vi "Decode scancodes into ascii.vi"(2 "PlatMods":T1, 3 "Mods":cluster{"Num Pad":bool, "Menu Key":bool}, 4 "ScanCode":i16) -> (0 "Numeric":i16, 1 "String":string)   [LabVIEW 2013]
doc: "Decode scanscodes into ascii.vi takes the scancode, mods, and platmods to index a case structure that outputs the ASCII value and the numeric value of the ASCII. Use this VI in the key up event if you want to programatically capture keystrikes.\n\nThe VI is easy to use, but tedious to write. There are 93 cases, each of which was experimentally verified."
panel:
  # "Select Help»Show Context Help and move the cursor \nover the VI icon to display help for this VI."
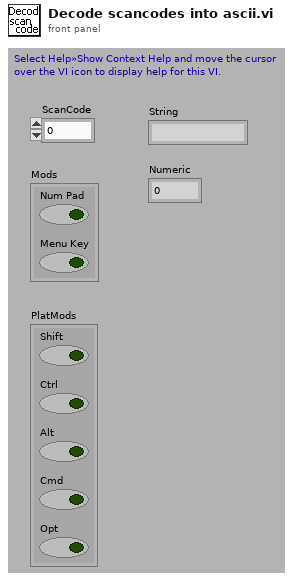
[diagram p1: front panel]
types:
  T1 = cluster{"Shift":bool, "Ctrl":bool, "Alt":bool, "Cmd":bool, "Opt":bool}
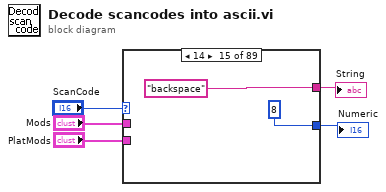
[diagram p0: block diagram]
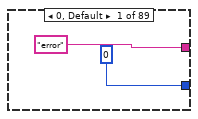
[diagram p2: hidden frame]
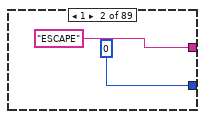
[diagram p3: hidden frame]
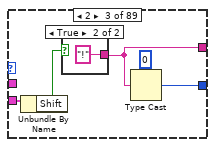
[diagram p4: hidden frame]
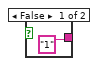
[diagram p5: hidden frame]
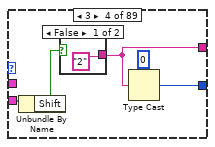
[diagram p6: hidden frame]
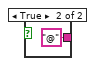
[diagram p7: hidden frame]
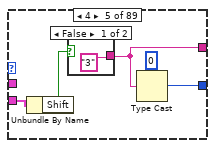
[diagram p8: hidden frame]
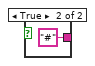
[diagram p9: hidden frame]
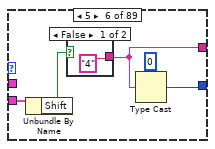
[diagram p10: hidden frame]
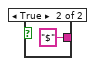
[diagram p11: hidden frame]
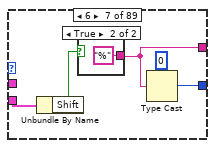
[diagram p12: hidden frame]
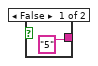
[diagram p13: hidden frame]
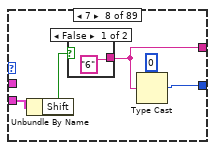
[diagram p14: hidden frame]
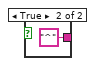
[diagram p15: hidden frame]
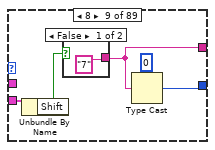
[diagram p16: hidden frame]
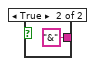
[diagram p17: hidden frame]
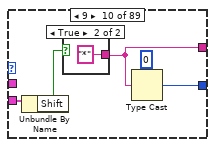
[diagram p18: hidden frame]
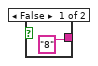
[diagram p19: hidden frame]
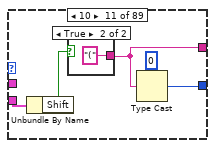
[diagram p20: hidden frame]
diagram:
  n1 = case shown="14" "ScanCode" {
    tunnel: ["error" "ESCAPE" w11 w19 w27 w35 w41 w45 w56 w63 w70 w76 w82 w87 "backspace" "tab" w100 w107 w114 w119 w126 w133 w140 w147 w154 w161 w168 w175 "Enter" "control" w188 w194 w202 w208 w215 w222 w229 w236 w243 w250 w256 w263 w272 w274 w282 w288 w295 w301 w308 w315 w322 w329 w336 w344 "RSHIFT" w355 "RSHIFT" "SPACE" "CAPSLOCK" "F1" "F2" "F3" "F4" "F5" "F6" "F7" "F8" "F9" "F10" "numlock" w389 w394 w403 w410 w419 w423 w431 w435 w443 w447 w455 w465 w476 w485 w491 w495 "left win key" "right win key" "select"] -> w2
    tunnel: "Mods" -> [_ _ _ _ _ _ _ _ _ _ _ _ _ _ _ _ _ _ _ _ _ _ _ _ _ _ _ _ _ _ _ _ _ _ _ _ _ _ _ _ _ _ _ _ _ _ _ _ _ _ _ _ _ _ _ w352 _ _ _ _ _ _ _ _ _ _ _ _ _ _ _ w393 w402 w412 _ w424 _ w436 _ w448 w457 w466 w473 w482 _ _ _ _ _]
    tunnel: "PlatMods" -> [_ _ w12 w18 w24 w32 w38 w47 w53 w60 w67 w73 w80 w89 _ _ w98 w105 w112 w120 w128 w134 w141 w149 w156 w163 w170 w177 _ _ w186 w193 w200 w207 w214 w221 w228 w235 w242 w249 w257 w264 _ w273 w283 w287 w294 w302 w309 w316 w323 w330 w337 w343 _ _ _ _ _ _ _ _ _ _ _ _ _ _ _ _ _ _ _ _ _ _ _ _ _ _ _ _ _ _ _ _ _ _ _]
    tunnel: [u8 0 u8 0 w13 w17 w28 w31 w42 w46 w52 w59 w66 w77 w81 w88 u8 8 u8 9 w99 w106 w113 w123 w127 w137 w144 w148 w155 w162 w169 w176 u8 0 u8 0 w187 w197 w201 w211 w218 w225 w232 w239 w246 w253 w260 w267 w270 w277 w281 w291 w298 w305 w312 w319 w326 w333 w340 w347 u8 0 w354 u8 0 u8 32 u8 0 u8 0 u8 0 u8 0 u8 0 u8 0 u8 0 u8 0 u8 0 u8 0 u8 0 u8 0 w390 w392 w404 w411 w420 w422 w432 w434 w444 w446 w456 w464 w475 w484 w492 w494 u8 0 u8 0 u8 0] -> w5
    frame 0, Default {
    }
    frame 1 {
    }
    frame 2 {
      n2 = Unbundle By Name(w12) -> ("Shift"=w10:bool)
      n3 = case shown="True" w10 {
        tunnel: ["1" "!"] -> w11
        frame False {
        }
        frame True {
        }
      }
      n4 = Type Cast(type=u8 0, x=w11) -> (*(type *) &x=w13:u8)
    }
    frame 3 {
      n5 = Unbundle By Name(w18) -> ("Shift"=w20:bool)
      n6 = case shown="False" w20 {
        tunnel: ["2" "@"] -> w19
        frame False {
        }
        frame True {
        }
      }
      n7 = Type Cast(type=u8 0, x=w19) -> (*(type *) &x=w17:u8)
    }
    frame 4 {
      n8 = Unbundle By Name(w24) -> ("Shift"=w25:bool)
      n9 = case shown="False" w25 {
        tunnel: ["3" "#"] -> w27
        frame False {
        }
        frame True {
        }
      }
      n10 = Type Cast(type=u8 0, x=w27) -> (*(type *) &x=w28:u8)
    }
    frame 5 {
      n11 = Unbundle By Name(w32) -> ("Shift"=w33:bool)
      n12 = case shown="False" w33 {
        tunnel: ["4" "$"] -> w35
        frame False {
        }
        frame True {
        }
      }
      n13 = Type Cast(type=u8 0, x=w35) -> (*(type *) &x=w31:u8)
    }
    frame 6 {
      n14 = Unbundle By Name(w38) -> ("Shift"=w39:bool)
      n15 = case shown="True" w39 {
        tunnel: ["5" "%"] -> w41
        frame False {
        }
        frame True {
        }
      }
      n16 = Type Cast(type=u8 0, x=w41) -> (*(type *) &x=w42:u8)
    }
    frame 7 {
      n17 = Unbundle By Name(w47) -> ("Shift"=w49:bool)
      n18 = case shown="False" w49 {
        tunnel: ["6" "^"] -> w45
        frame False {
        }
        frame True {
        }
      }
      n19 = Type Cast(type=u8 0, x=w45) -> (*(type *) &x=w46:u8)
    }
    frame 8 {
      n20 = Unbundle By Name(w53) -> ("Shift"=w55:bool)
      n21 = case shown="False" w55 {
        tunnel: ["7" "&"] -> w56
        frame False {
        }
        frame True {
        }
      }
      n22 = Type Cast(type=u8 0, x=w56) -> (*(type *) &x=w52:u8)
    }
    frame 9 {
      n23 = Unbundle By Name(w60) -> ("Shift"=w61:bool)
      n24 = case shown="True" w61 {
        tunnel: ["8" "*"] -> w63
        frame False {
        }
        frame True {
        }
      }
      n25 = Type Cast(type=u8 0, x=w63) -> (*(type *) &x=w59:u8)
    }
    frame 10 {
      n26 = Unbundle By Name(w67) -> ("Shift"=w69:bool)
      n27 = case shown="True" w69 {
        tunnel: ["9" "("] -> w70
        frame False {
        }
        frame True {
        }
      }
      n28 = Type Cast(type=u8 0, x=w70) -> (*(type *) &x=w66:u8)
    }
    frame 11 {
      n29 = Unbundle By Name(w73) -> ("Shift"=w74:bool)
      n30 = case shown="False" w74 {
        tunnel: ["0" ")"] -> w76
        frame False {
        }
        frame True {
        }
      }
      n31 = Type Cast(type=u8 0, x=w76) -> (*(type *) &x=w77:u8)
    }
    frame 12 {
      n32 = Unbundle By Name(w80) -> ("Shift"=w84:bool)
      n33 = case shown="False" w84 {
        tunnel: ["-" "_"] -> w82
        frame False {
        }
        frame True {
        }
      }
      n34 = Type Cast(type=u8 0, x=w82) -> (*(type *) &x=w81:u8)
    }
    frame 13 {
      n35 = Unbundle By Name(w89) -> ("Shift"=w90:bool)
      n36 = case shown="False" w90 {
        tunnel: ["=" "+"] -> w87
        frame False {
        }
        frame True {
        }
      }
      n37 = Type Cast(type=u8 0, x=w87) -> (*(type *) &x=w88:u8)
    }
    frame 14 {
    }
    frame 15 {
    }
    frame 16 {
      n38 = Unbundle By Name(w98) -> ("Shift"=w102:bool)
      n39 = case shown="True" w102 {
        tunnel: ["q" "Q"] -> w100
        frame False {
        }
        frame True {
        }
      }
      n40 = Type Cast(type=u8 0, x=w100) -> (*(type *) &x=w99:u8)
    }
    frame 17 {
      n41 = Unbundle By Name(w105) -> ("Shift"=w108:bool)
      n42 = case shown="True" w108 {
        tunnel: ["w" "W"] -> w107
        frame False {
        }
        frame True {
        }
      }
      n43 = Type Cast(type=u8 0, x=w107) -> (*(type *) &x=w106:u8)
    }
    frame 18 {
      n44 = Unbundle By Name(w112) -> ("Shift"=w116:bool)
      n45 = case shown="True" w116 {
        tunnel: ["e" "E"] -> w114
        frame False {
        }
        frame True {
        }
      }
      n46 = Type Cast(type=u8 0, x=w114) -> (*(type *) &x=w113:u8)
    }
    frame 19 {
      n47 = Unbundle By Name(w120) -> ("Shift"=w121:bool)
      n48 = case shown="True" w121 {
        tunnel: ["r" "R"] -> w119
        frame False {
        }
        frame True {
        }
      }
      n49 = Type Cast(type=u8 0, x=w119) -> (*(type *) &x=w123:u8)
    }
    frame 20 {
      n50 = Unbundle By Name(w128) -> ("Shift"=w129:bool)
      n51 = case shown="True" w129 {
        tunnel: ["t" "T"] -> w126
        frame False {
        }
        frame True {
        }
      }
      n52 = Type Cast(type=u8 0, x=w126) -> (*(type *) &x=w127:u8)
    }
    frame 21 {
      n53 = Unbundle By Name(w134) -> ("Shift"=w135:bool)
      n54 = case shown="True" w135 {
        tunnel: ["y" "Y"] -> w133
        frame False {
        }
        frame True {
        }
      }
      n55 = Type Cast(type=u8 0, x=w133) -> (*(type *) &x=w137:u8)
    }
    frame 22 {
      n56 = Unbundle By Name(w141) -> ("Shift"=w143:bool)
      n57 = case shown="True" w143 {
        tunnel: ["u" "U"] -> w140
        frame False {
        }
        frame True {
        }
      }
      n58 = Type Cast(type=u8 0, x=w140) -> (*(type *) &x=w144:u8)
    }
    frame 23 {
      n59 = Unbundle By Name(w149) -> ("Shift"=w150:bool)
      n60 = case shown="True" w150 {
        tunnel: ["i" "I"] -> w147
        frame False {
        }
        frame True {
        }
      }
      n61 = Type Cast(type=u8 0, x=w147) -> (*(type *) &x=w148:u8)
    }
    frame 24 {
      n62 = Unbundle By Name(w156) -> ("Shift"=w158:bool)
      n63 = case shown="True" w158 {
        tunnel: ["o" "O"] -> w154
        frame False {
        }
        frame True {
        }
      }
      n64 = Type Cast(type=u8 0, x=w154) -> (*(type *) &x=w155:u8)
    }
    frame 25 {
      n65 = Unbundle By Name(w163) -> ("Shift"=w165:bool)
      n66 = case shown="True" w165 {
        tunnel: ["p" "P"] -> w161
        frame False {
        }
        frame True {
        }
      }
      n67 = Type Cast(type=u8 0, x=w161) -> (*(type *) &x=w162:u8)
    }
    frame 26 {
      n68 = Unbundle By Name(w170) -> ("Shift"=w171:bool)
      n69 = case shown="True" w171 {
        tunnel: ["[" "{"] -> w168
        frame False {
        }
        frame True {
        }
      }
      n70 = Type Cast(type=u8 0, x=w168) -> (*(type *) &x=w169:u8)
    }
    frame 27 {
      n71 = Unbundle By Name(w177) -> ("Shift"=w179:bool)
      n72 = case shown="False" w179 {
        tunnel: ["}" "P"] -> w175
        frame False {
        }
        frame True {
        }
      }
      n73 = Type Cast(type=u8 0, x=w175) -> (*(type *) &x=w176:u8)
    }
    frame 28 {
    }
    frame 29 {
    }
    frame 30 {
      n74 = Unbundle By Name(w186) -> ("Shift"=w189:bool)
      n75 = case shown="True" w189 {
        tunnel: ["a" "A"] -> w188
        frame False {
        }
        frame True {
        }
      }
      n76 = Type Cast(type=u8 0, x=w188) -> (*(type *) &x=w187:u8)
    }
    frame 31 {
      n77 = Unbundle By Name(w193) -> ("Shift"=w196:bool)
      n78 = case shown="True" w196 {
        tunnel: ["s" "S"] -> w194
        frame False {
        }
        frame True {
        }
      }
      n79 = Type Cast(type=u8 0, x=w194) -> (*(type *) &x=w197:u8)
    }
    frame 32 {
      n80 = Unbundle By Name(w200) -> ("Shift"=w203:bool)
      n81 = case shown="True" w203 {
        tunnel: ["d" "D"] -> w202
        frame False {
        }
        frame True {
        }
      }
      n82 = Type Cast(type=u8 0, x=w202) -> (*(type *) &x=w201:u8)
    }
    frame 33 {
      n83 = Unbundle By Name(w207) -> ("Shift"=w209:bool)
      n84 = case shown="True" w209 {
        tunnel: ["f" "F"] -> w208
        frame False {
        }
        frame True {
        }
      }
      n85 = Type Cast(type=u8 0, x=w208) -> (*(type *) &x=w211:u8)
    }
    frame 34 {
      n86 = Unbundle By Name(w214) -> ("Shift"=w217:bool)
      n87 = case shown="True" w217 {
        tunnel: ["g" "G"] -> w215
        frame False {
        }
        frame True {
        }
      }
      n88 = Type Cast(type=u8 0, x=w215) -> (*(type *) &x=w218:u8)
    }
    frame 35 {
      n89 = Unbundle By Name(w221) -> ("Shift"=w223:bool)
      n90 = case shown="True" w223 {
        tunnel: ["h" "H"] -> w222
        frame False {
        }
        frame True {
        }
      }
      n91 = Type Cast(type=u8 0, x=w222) -> (*(type *) &x=w225:u8)
    }
    frame 36 {
      n92 = Unbundle By Name(w228) -> ("Shift"=w231:bool)
      n93 = case shown="True" w231 {
        tunnel: ["j" "J"] -> w229
        frame False {
        }
        frame True {
        }
      }
      n94 = Type Cast(type=u8 0, x=w229) -> (*(type *) &x=w232:u8)
    }
    frame 37 {
      n95 = Unbundle By Name(w235) -> ("Shift"=w238:bool)
      n96 = case shown="True" w238 {
        tunnel: ["k" "K"] -> w236
        frame False {
        }
        frame True {
        }
      }
      n97 = Type Cast(type=u8 0, x=w236) -> (*(type *) &x=w239:u8)
    }
    frame 38 {
      n98 = Unbundle By Name(w242) -> ("Shift"=w244:bool)
      n99 = case shown="True" w244 {
        tunnel: ["l" "L"] -> w243
        frame False {
        }
        frame True {
        }
      }
      n100 = Type Cast(type=u8 0, x=w243) -> (*(type *) &x=w246:u8)
    }
    frame 39 {
      n101 = Unbundle By Name(w249) -> ("Shift"=w252:bool)
      n102 = case shown="True" w252 {
        tunnel: [";" ":"] -> w250
        frame False {
        }
        frame True {
        }
      }
      n103 = Type Cast(type=u8 0, x=w250) -> (*(type *) &x=w253:u8)
    }
    frame 40 {
      n104 = Unbundle By Name(w257) -> ("Shift"=w258:bool)
      n105 = case shown="True" w258 {
        tunnel: ["'" "\""] -> w256
        frame False {
        }
        frame True {
        }
      }
      n106 = Type Cast(type=u8 0, x=w256) -> (*(type *) &x=w260:u8)
    }
    frame 41 {
      n107 = Unbundle By Name(w264) -> ("Shift"=w266:bool)
      n108 = case shown="True" w266 {
        tunnel: ["`" "~"] -> w263
        frame False {
        }
        frame True {
        }
      }
      n109 = Type Cast(type=u8 0, x=w263) -> (*(type *) &x=w267:u8)
    }
    frame 42 {
      w272 = "LSHIFT"
      n110 = Type Cast(type=u8 0, x=w272) -> (*(type *) &x=w270:u8)
    }
    frame 43 {
      n111 = Unbundle By Name(w273) -> ("Shift"=w276:bool)
      n112 = case shown="True" w276 {
        tunnel: [";" ":"] -> w274
        frame False {
        }
        frame True {
        }
      }
      n113 = Type Cast(type=u8 0, x=w274) -> (*(type *) &x=w277:u8)
    }
    frame 44 {
      n114 = Unbundle By Name(w283) -> ("Shift"=w284:bool)
      n115 = case shown="False" w284 {
        tunnel: ["z" "Z"] -> w282
        frame False {
        }
        frame True {
        }
      }
      n116 = Type Cast(type=u8 0, x=w282) -> (*(type *) &x=w281:u8)
    }
    frame 45 {
      n117 = Unbundle By Name(w287) -> ("Shift"=w290:bool)
      n118 = case shown="False" w290 {
        tunnel: ["x" "X"] -> w288
        frame False {
        }
        frame True {
        }
      }
      n119 = Type Cast(type=u8 0, x=w288) -> (*(type *) &x=w291:u8)
    }
    frame 46 {
      n120 = Unbundle By Name(w294) -> ("Shift"=w296:bool)
      n121 = case shown="False" w296 {
        tunnel: ["c" "C"] -> w295
        frame False {
        }
        frame True {
        }
      }
      n122 = Type Cast(type=u8 0, x=w295) -> (*(type *) &x=w298:u8)
    }
    frame 47 {
      n123 = Unbundle By Name(w302) -> ("Shift"=w304:bool)
      n124 = case shown="False" w304 {
        tunnel: ["v" "V"] -> w301
        frame False {
        }
        frame True {
        }
      }
      n125 = Type Cast(type=u8 0, x=w301) -> (*(type *) &x=w305:u8)
    }
    frame 48 {
      n126 = Unbundle By Name(w309) -> ("Shift"=w310:bool)
      n127 = case shown="False" w310 {
        tunnel: ["b" "B"] -> w308
        frame False {
        }
        frame True {
        }
      }
      n128 = Type Cast(type=u8 0, x=w308) -> (*(type *) &x=w312:u8)
    }
    frame 49 {
      n129 = Unbundle By Name(w316) -> ("Shift"=w318:bool)
      n130 = case shown="False" w318 {
        tunnel: ["n" "N"] -> w315
        frame False {
        }
        frame True {
        }
      }
      n131 = Type Cast(type=u8 0, x=w315) -> (*(type *) &x=w319:u8)
    }
    frame 50 {
      n132 = Unbundle By Name(w323) -> ("Shift"=w324:bool)
      n133 = case shown="False" w324 {
        tunnel: ["m" "M"] -> w322
        frame False {
        }
        frame True {
        }
      }
      n134 = Type Cast(type=u8 0, x=w322) -> (*(type *) &x=w326:u8)
    }
    frame 51 {
      n135 = Unbundle By Name(w330) -> ("Shift"=w331:bool)
      n136 = case shown="False" w331 {
        tunnel: ["," "<"] -> w329
        frame False {
        }
        frame True {
        }
      }
      n137 = Type Cast(type=u8 0, x=w329) -> (*(type *) &x=w333:u8)
    }
    frame 52 {
      n138 = Unbundle By Name(w337) -> ("Shift"=w339:bool)
      n139 = case shown="False" w339 {
        tunnel: ["." ">"] -> w336
        frame False {
        }
        frame True {
        }
      }
      n140 = Type Cast(type=u8 0, x=w336) -> (*(type *) &x=w340:u8)
    }
    frame 53 {
      n141 = Unbundle By Name(w343) -> ("Shift"=w345:bool)
      n142 = case shown="False" w345 {
        tunnel: ["/" "?"] -> w344
        frame False {
        }
        frame True {
        }
      }
      n143 = Type Cast(type=u8 0, x=w344) -> (*(type *) &x=w347:u8)
    }
    frame 54 {
    }
    frame 55 {
      n144 = Unbundle By Name(w352) -> ("Num Pad"=w353:bool)
      n145 = case shown="True" w353 {
        tunnel: [-1 w359] -> w354
        tunnel: ["PRINTSCREEN" w358] -> w355
        frame False {
        }
        frame True {
          w358 = "/"
          n146 = Type Cast(type=u8 0, x=w358) -> (*(type *) &x=w359:u8)
        }
      }
    }
    frame 56 {
    }
    frame 57 {
    }
    frame 58 {
    }
    frame 59 {
    }
    frame 60 {
    }
    frame 61 {
    }
    frame 62 {
    }
    frame 63 {
    }
    frame 64 {
    }
    frame 65 {
    }
    frame 66 {
    }
    frame 67 {
    }
    frame 68 {
    }
    frame 69 {
    }
    frame 70 {
      w389 = "error"
      n147 = Type Cast(type=u8 0, x=w389) -> (*(type *) &x=w390:u8)
    }
    frame 71 {
      n148 = Unbundle By Name(w393) -> ("Num Pad"=w395:bool)
      n149 = case shown="True" w395 {
        tunnel: [-1 w399] -> w392
        tunnel: ["HOME" w398] -> w394
        frame False {
        }
        frame True {
          w398 = "7"
          n150 = Type Cast(type=u8 0, x=w398) -> (*(type *) &x=w399:u8)
        }
      }
    }
    frame 72 {
      n151 = Unbundle By Name(w402) -> ("Num Pad"=w401:bool)
      n152 = case shown="False" w401 {
        tunnel: [-1 w408] -> w404
        tunnel: ["UP" w407] -> w403
        frame False {
        }
        frame True {
          w407 = "8"
          n153 = Type Cast(type=u8 0, x=w407) -> (*(type *) &x=w408:u8)
        }
      }
    }
    frame 73 {
      n154 = Unbundle By Name(w412) -> ("Num Pad"=w413:bool)
      n155 = case shown="True" w413 {
        tunnel: [-1 w417] -> w411
        tunnel: ["PAGEUP" w416] -> w410
        frame False {
        }
        frame True {
          w416 = "9"
          n156 = Type Cast(type=u8 0, x=w416) -> (*(type *) &x=w417:u8)
        }
      }
    }
    frame 74 {
      w419 = "-"
      n157 = Type Cast(type=u8 0, x=w419) -> (*(type *) &x=w420:u8)
    }
    frame 75 {
      n158 = Unbundle By Name(w424) -> ("Num Pad"=w425:bool)
      n159 = case shown="True" w425 {
        tunnel: [-1 w429] -> w422
        tunnel: ["LEFT" w428] -> w423
        frame False {
        }
        frame True {
          w428 = "4"
          n160 = Type Cast(type=u8 0, x=w428) -> (*(type *) &x=w429:u8)
        }
      }
    }
    frame 76 {
      w431 = "5"
      n161 = Type Cast(type=u8 0, x=w431) -> (*(type *) &x=w432:u8)
    }
    frame 77 {
      n162 = Unbundle By Name(w436) -> ("Num Pad"=w437:bool)
      n163 = case shown="True" w437 {
        tunnel: [-1 w441] -> w434
        tunnel: ["RIGHT" w440] -> w435
        frame False {
        }
        frame True {
          w440 = "6"
          n164 = Type Cast(type=u8 0, x=w440) -> (*(type *) &x=w441:u8)
        }
      }
    }
    frame 78 {
      w443 = "+"
      n165 = Type Cast(type=u8 0, x=w443) -> (*(type *) &x=w444:u8)
    }
    frame 79 {
      n166 = Unbundle By Name(w448) -> ("Num Pad"=w449:bool)
      n167 = case shown="False" w449 {
        tunnel: [-1 w453] -> w446
        tunnel: ["END" w452] -> w447
        frame False {
        }
        frame True {
          w452 = "1"
          n168 = Type Cast(type=u8 0, x=w452) -> (*(type *) &x=w453:u8)
        }
      }
    }
    frame 80 {
      n169 = Unbundle By Name(w457) -> ("Num Pad"=w458:bool)
      n170 = case shown="True" w458 {
        tunnel: [-1 w462] -> w456
        tunnel: ["DOWN" w461] -> w455
        frame False {
        }
        frame True {
          w461 = "2"
          n171 = Type Cast(type=u8 0, x=w461) -> (*(type *) &x=w462:u8)
        }
      }
    }
    frame 81 {
      n172 = Unbundle By Name(w466) -> ("Num Pad"=w467:bool)
      n173 = case shown="False" w467 {
        tunnel: [-1 w471] -> w464
        tunnel: ["PAGEDOWN" w470] -> w465
        frame False {
        }
        frame True {
          w470 = "3"
          n174 = Type Cast(type=u8 0, x=w470) -> (*(type *) &x=w471:u8)
        }
      }
    }
    frame 82 {
      n175 = Unbundle By Name(w473) -> ("Num Pad"=w474:bool)
      n176 = case shown="True" w474 {
        tunnel: [-1 w480] -> w475
        tunnel: ["INSERT" w479] -> w476
        frame False {
        }
        frame True {
          w479 = "0"
          n177 = Type Cast(type=u8 0, x=w479) -> (*(type *) &x=w480:u8)
        }
      }
    }
    frame 83 {
      n178 = Unbundle By Name(w482) -> ("Num Pad"=w483:bool)
      n179 = case shown="True" w483 {
        tunnel: [-1 w489] -> w484
        tunnel: ["DELETE" w488] -> w485
        frame False {
        }
        frame True {
          w488 = "."
          n180 = Type Cast(type=u8 0, x=w488) -> (*(type *) &x=w489:u8)
        }
      }
    }
    frame 87 {
      w491 = "F11"
      n181 = Type Cast(type=u8 0, x=w491) -> (*(type *) &x=w492:u8)
    }
    frame 88 {
      w495 = "F12"
      n182 = Type Cast(type=u8 0, x=w495) -> (*(type *) &x=w494:u8)
    }
    frame 91 {
    }
    frame 92 {
    }
    frame 93 {
    }
  }
  "Numeric" <- w5
  "String" <- w2
